vi "PID Output Rate Limiter.vi"(7 "reinitialize? (F)":bool, 8 "dt (s)":dbl=-1.0 format="%.2f", 10 "input (controller output)":dbl format="%.2f", 11 "PID Output Rate Limiter in":refnum<class "PID Output Rate Limiter.lvclass">) -> (0 "dt (s) out":dbl, 2 "output":dbl format="%.2f", 3 "PID Output Rate Limiter out":refnum<class "PID Output Rate Limiter.lvclass">)   [LabVIEW 2019, in "control.lvlib" / "PID Output Rate Limiter.lvclass"]
uses:
  PID Output Rate Limiter.lvclass
  D:/my_projects/projects/Algorithms/Labview/19/Reg/PID/PID Timing Estimation/PID Timing Estimation.lvclass
  PID Timing Estimation/PID Timing Estimation.lvclass/PID Timing Estimation.ctl
  PID Output Rate Limiter.lvclass/PID Output Rate Limiter.ctl
  PID Timing Estimation/PID Timing Estimation.lvclass
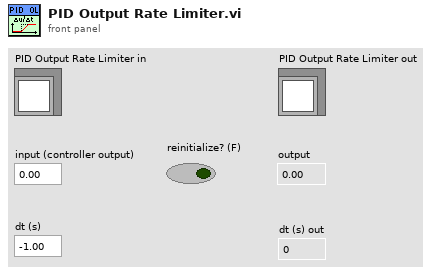
[diagram p1: front panel]
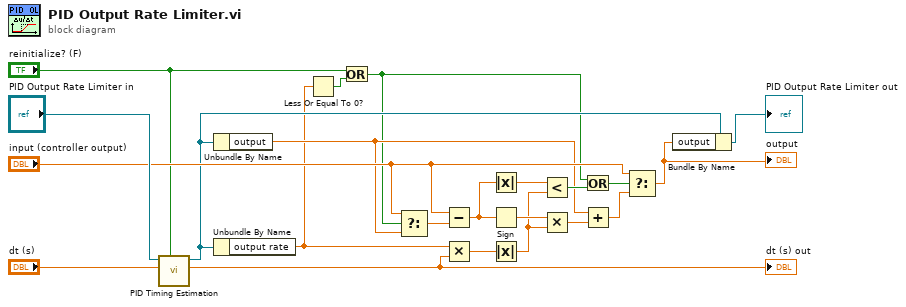
[diagram p0: block diagram]
diagram:
  n1 = call "PID Timing Estimation.vi"("R"="reinitialize? (F)", "dt (s) in"="dt (s)", "PID Timing Estimation in"="PID Output Rate Limiter in") -> ("dt (s) out"=w5:dbl, "PID Timing Estimation out"=w6:refnum<class "PID Output Rate Limiter.lvclass">)  [unwired: 7 in]
  "dt (s) out" <- w5
  n2 = Unbundle By Name(w6) -> ("output"=w7:dbl)
  n3 = Unbundle By Name(w6) -> ("output rate"=w3:dbl)
  n4 = Less Or Equal To 0?(x=w3) -> (x <= 0?=w2:bool)
  n5 = Or(x="reinitialize? (F)", y=w2) -> (x .or. y?=w1:bool)
  n6 = Select(t="input (controller output)", s=w1, f=w7) -> (s? t:f=w12:dbl)
  n7 = Subtract(x="input (controller output)", y=w12) -> (x-y=w15:dbl)
  n8 = Multiply(x=w3, y=w5) -> (x*y=w17:dbl)
  n9 = Absolute Value(x=w15) -> (abs(x)=w11:dbl)
  n10 = Sign(1:w15) -> (0:w13:dbl)
  n11 = Absolute Value(x=w17) -> (abs(x)=w10:dbl)
  n12 = Less?(x=w11, y=w10) -> (x < y?=w16:bool)
  n13 = Multiply(x=w13, y=w10) -> (x*y=w8:dbl)
  n14 = Or(x=w1, y=w16) -> (x .or. y?=w9:bool)
  n15 = Add(x=w7, y=w8) -> (x+y=w14:dbl)
  n16 = Select(t="input (controller output)", s=w9, f=w14) -> (s? t:f=w20:dbl)
  "output" <- w20
  n17 = Bundle By Name(cluster=w6, "output"=w20) -> (→"PID Output Rate Limiter out":refnum<class "PID Output Rate Limiter.lvclass">)
